vi "Sweep Config.vi"(0 "VISA resource name":refnum<visa-resource-name>, 1 "Start Value":dbl, 2 "End Value":dbl, 3 "Points (1)":u32=1 min=1, 5 "Node In":string, 7 "Channel (Channel A)":T2, 9 "Sweep Type":T1(ring), 11 "error in":errorcluster, 12 "Sweep Mode (F: Disable)":bool, 13 "Limit (0.1)":dbl=0.1, 14 "Sweep List":string) -> (4 "VISA resource name out":refnum<visa-resource-name>, 6 "Node Out":string, 10 "Command String":string, 15 "error out":errorcluster)   [LabVIEW 2009, in "Keithley 2600 Series.lvlib"]
doc: "This VI configures a sweep.\n\nUse this VI to enable/disable sweeps and to configure the sweep type and sweep levels.\n\n<b>Functions and Attributes Used</b>\nsmuX.trigger.source.action\nsmuX.trigger.source.linearY()\nsmuX.trigger.source.logY()\nsmuX.trigger.source.listY()\nsmuX.trigger.source.limitY\nsmuX.trigger.source.limiti"
uses:
  <instrlib>/Keithley 2600 Series/Keithley 2600 Series.lvlib
  <instrlib>/Keithley 2600 Series/Public/Channel.ctl
  <instrlib>/Keithley 2600 Series/Private/GlobalVariables.vi
panel:
  in  "Limit Current Mode Off (F:Disable)":bool
  # "(c) 2011 Keithley Instruments, Inc.  ALL RIGHTS RESERVED."
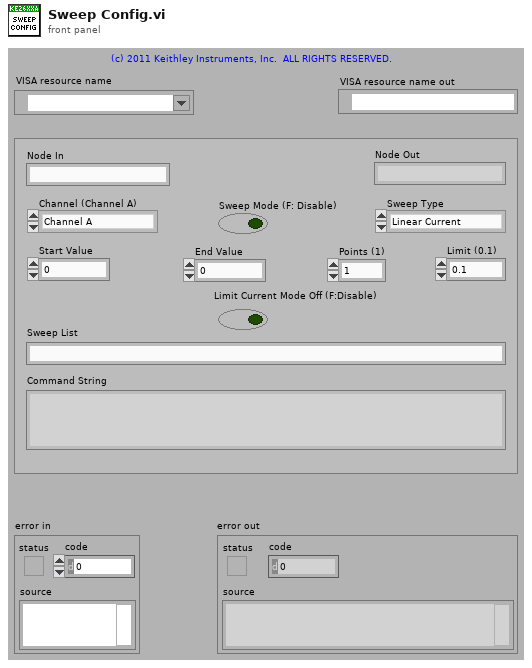
[diagram p1: front panel]
types:
  T1 = enum16{"Linear Current", "Linear Voltage", "Logarithimic Current", "Logarithimic Voltage", "List Current", "List Voltage"}
  T2 = typedef "Keithley 2600 Series.lvlib/Channel.ctl" = enum32{"Channel A", "Channel B"}
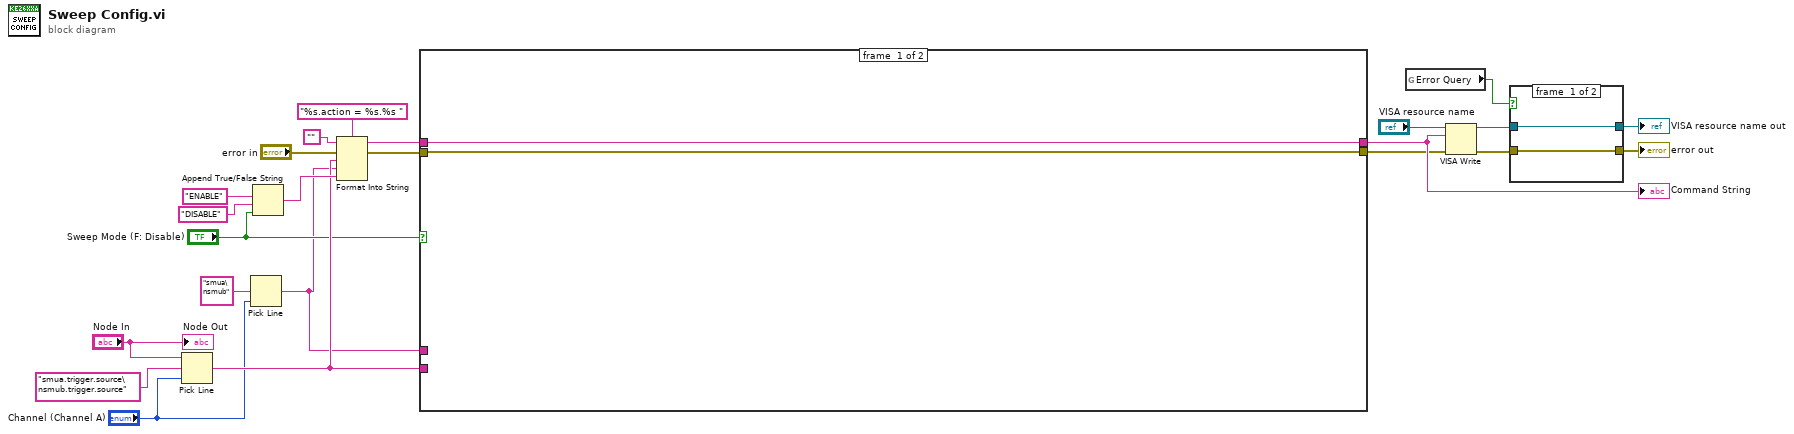
[diagram p0: block diagram]
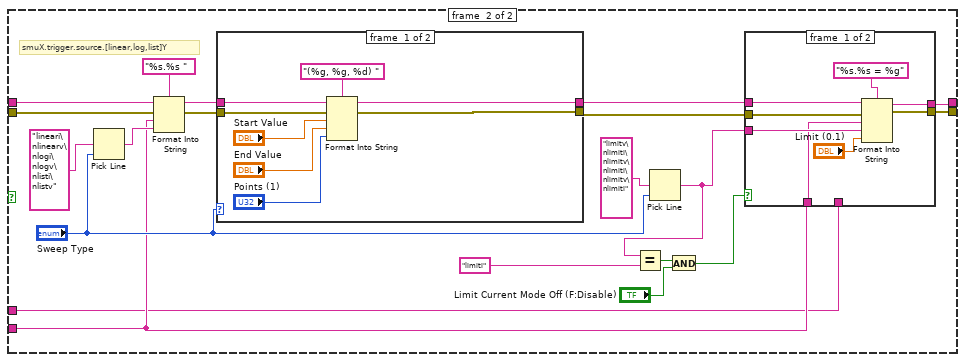
[diagram p2: hidden frame]
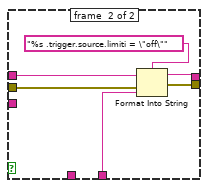
[diagram p3: hidden frame]
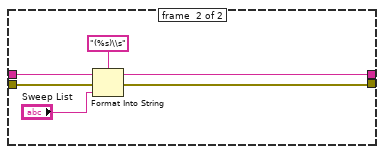
[diagram p4: hidden frame]
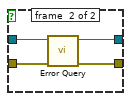
[diagram p5: hidden frame]
diagram:
  n1 = Pick Line(string ("")="Node In", multi-line string="smua.trigger.source\nsmub.trigger.source", line index="Channel (Channel A)") -> (output string=w6:string)
  n2 = Pick Line(multi-line string="smua\nsmub", line index="Channel (Channel A)") -> (output string=w1:string)  [unwired: 1 out]
  n3 = Append True/False String(1:"Sweep Mode (F: Disable)", 2:"DISABLE" ("false string"), 3:"ENABLE" ("true string")) -> (0:w13:string)  [unwired: 1 out]
  n4 = Format Into String(format string="%s.action = %s.%s ", initial string="", error in="error in", w6, w1, w13) -> (resulting string=w8:string, error out=w7:errorcluster)
  n5 = case shown="True" "Sweep Mode (F: Disable)" {
    tunnel: [w25 w42] -> w15
    tunnel: [w24 w41] -> w14
    tunnel: w8 -> [w25 w34]
    tunnel: w7 -> [w24 w33]
    tunnel: w6 -> [_ w32]
    tunnel: w1 -> [_ w26]
    frame #0 {
    }
    frame #1 {
      # "smuX.trigger.source.[linear,log,list]Y"
      n6 = Pick Line(multi-line string="lineari\nlinearv\nlogi\nlogv\nlisti\nlistv", line index="Sweep Type") -> (output string=w35:string)  [unwired: 1 out]
      n7 = Format Into String(format string="%s.%s ", initial string=w34, error in=w33, w32, w35) -> (resulting string=w37:string, error out=w36:errorcluster)
      n8 = case shown="\"Linear Current\"..\"Logarithimic Voltage\"" "Sweep Type" {
        tunnel: w37 -> [w66 w72]
        tunnel: w36 -> [w65 w71]
        tunnel: [w61 w69] -> w45
        tunnel: [w60 w68] -> w44
        frame #0 {
          n9 = Format Into String(format string="(%g, %g, %d) ", initial string=w66, error in=w65, "Start Value", "End Value", "Points (1)") -> (resulting string=w61:string, error out=w60:errorcluster)
        }
        frame #1 {
          n10 = Format Into String(format string="(%s)\\s", initial string=w72, error in=w71, "Sweep List") -> (resulting string=w69:string, error out=w68:errorcluster)
        }
      }
      n11 = Pick Line(multi-line string="limitv\nlimiti\nlimitv\nlimiti\nlimitv\nlimiti", line index="Sweep Type") -> (output string=w29:string)  [unwired: 1 out]
      n12 = Equal?(x=w29, y="limiti") -> (x = y?=w30:bool)
      n13 = And(x=w30, y="Limit Current Mode Off (F:Disable)") -> (x .and. y?=w31:bool)
      n14 = case shown="False" w31 {
        tunnel: w45 -> [w53 w57]
        tunnel: w44 -> [w52 w55]
        tunnel: w29 -> [w50 _]
        tunnel: [w48 w59] -> w42
        tunnel: [w47 w54] -> w41
        tunnel: w32 -> [w46 _]
        tunnel: w26 -> [_ w58]
        frame #0 {
          n15 = Format Into String(format string="%s.%s = %g", initial string=w53, error in=w52, w46, w50, "Limit (0.1)") -> (resulting string=w48:string, error out=w47:errorcluster)
        }
        frame #1 {
          n16 = Format Into String(format string="%s .trigger.source.limiti = \"off\"", initial string=w57, error in=w55, w58) -> (resulting string=w59:string, error out=w54:errorcluster)
        }
      }
    }
  }
  "Command String" <- w15
  n17 = global read "GlobalVariables.vi" "Error Query"() -> (w20:bool)
  n18 = VISA Write(VISA resource name="VISA resource name", write buffer=w15, error in (no error)=w14) -> (VISA resource name out=w19:refnum<visa-resource-name>, error out=w18:errorcluster)  [unwired: 1 out]
  n19 = case shown="True" w20 {
    tunnel: w19 -> [w75 w79]
    tunnel: w18 -> [w74 w78]
    tunnel: [w75 w77] -> w17
    tunnel: [w74 w76] -> w16
    frame #0 {
    }
    frame #1 {
      n20 = call <instrlib>:"Error Query.vi"("error in (no error)"=w78, "VISA resource name"=w79) -> ("error out"=w76:errorcluster, "VISA resource name out"=w77:refnum<visa-resource-name>)  [unwired: 8 out]
    }
  }
  "VISA resource name out" <- w17
  "error out" <- w16
  "Node Out" <- "Node In"
